vi "ble_read_by_service_characteristic.vi"(5 "Characteristic UUID":string, 6 "Connection Status":T1={"MAC Address"="", "cnx handle"=0, "cnx flags"=0, "Address Type"=125, "Connection Interval (ms)"=125, "Timeout(ms)"=125, "Latency"=0, "bonding handle"=0} {"Address Type" items=["Public", "Random"]}, 7 "Service UUID":string, 8 "error in (no error)":errorcluster, 9 "Read long?(T)":bool=TRUE, 10 "Handle table":string[][](array[string]), 11 "COM Bluegiga in":refnum<visa-resource-name>) -> (0 "error out":errorcluster, 1 "attribute value":u8[](array[numeric]), 2 "payload":u8[](array[numeric]), 3 "COM Bluegiga out":refnum<visa-resource-name>)   [LabVIEW 2013]
uses:
  type_def/connection_status_bundle.ctl
  type_def/address_type.ctl
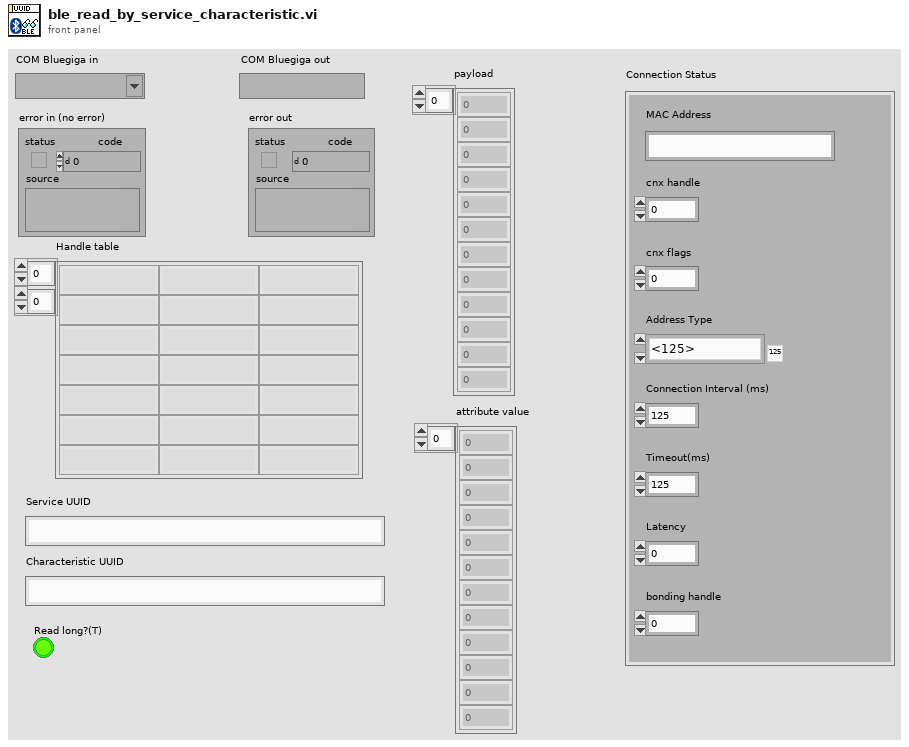
[diagram p1: front panel]
types:
  T1 = typedef "connection_status_bundle.ctl" = cluster{"MAC Address":string, "cnx handle":u8, "cnx flags":u8, "Address Type":T2, "Connection Interval (ms)":u16, "Timeout(ms)":u16, "Latency":u16, "bonding handle":u8}
  T2 = typedef "address_type.ctl" = u8
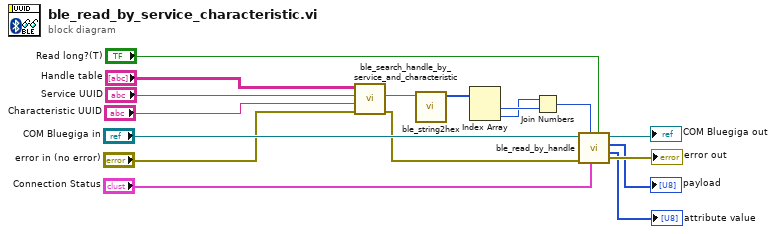
[diagram p0: block diagram]
diagram:
  n1 = call "ble_search_handle_by_service_and_characteristic.vi"("error in (no error)"="error in (no error)", "Characteristic UUID"="Characteristic UUID", "Service UUID"="Service UUID", "Handle table"="Handle table") -> ("error out"=w6:errorcluster, "Handle"=w3:string)  [unwired: 6 in]
  n2 = call "ble_string2hex.vi"("HEX string IN"=w3) -> ("Byte Array IN (index0 LS byte)"=w4:u8[])  [unwired: 10 in]
  n3 = Index Array(array=w4) -> (element #1=w17:u8, element #2=w16:u8)  [unwired: 2 in]
  n4 = Join Numbers(hi=w16, lo=w17) -> ((hi.lo)=w15:u16)
  n5 = call "ble_read_by_handle.vi"("Read long?(T)"="Read long?(T)", "Connection Status"="Connection Status", "Handle"=w15, "error in (no error)"=w6, "COM Bluegiga in"="COM Bluegiga in") -> ("error out"=→"error out":errorcluster, "attribute value"=→"attribute value":u8[], "payload"=→"payload":u8[], "COM Bluegiga out"=→"COM Bluegiga out":refnum<visa-resource-name>)  [unwired: 3 in]
